vi "DAQmx_Put_Master_First.vi"(8 "error in (no error)":errorcluster, 11 "DAQmx in":refnum<class "DAQmx.lvclass">[](array[class])) -> (0 "error out":errorcluster, 3 "DAQmx out":refnum<class "DAQmx.lvclass">[](array[class]))   [LabVIEW 2020, in "DAQmx.lvclass"]
uses:
  DAQmx.lvclass
  DAQmx.lvclass/DAQmx.ctl
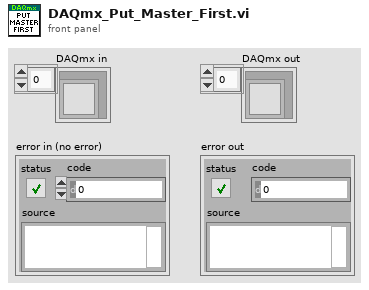
[diagram p1: front panel]
types:
  T1 = typedef "DAQmx.lvclass/DAQmx_Config.ctl" = cluster{"Buffer Size (S)":i32, "Master Slave":enum16{"MASTER", "SLAVE"}}
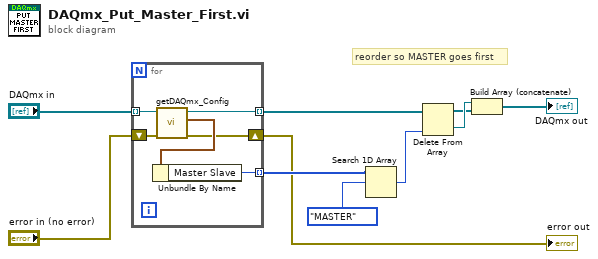
[diagram p0: block diagram]
diagram:
  # "reorder so MASTER goes first"
  n1 = for {
    tunnel: "DAQmx in" -> [w16] mode=indexing
    tunnel: [w14] -> w5 mode=indexing
    tunnel: [w13] -> w6 mode=indexing
    shift-right: [w11] -> w1
    shift-left: "error in (no error)" -> [w12]
    n2 = call "getDAQmx_Config.vi"("error in (no error)"=w12, "DAQmx in"=w16) -> ("error out"=w11:errorcluster, "DAQmx.Config"=w15:T1, "DAQmx out"=w13:refnum<class "DAQmx.lvclass">)  [unwired: 7 in]
    n3 = Unbundle By Name(w15) -> ("Master Slave"=w14:enum16{"MASTER", "SLAVE"})
  }
  "error out" <- w1
  n4 = Search 1D Array(1D array=w5, element=enum16{"MASTER", "SLAVE"}."MASTER" ("Master Slave")) -> (index of element=w3:i32)  [unwired: 1 in]
  n5 = Delete From Array(array=w6, index=w3) -> (deleted portion=w9:refnum<class "DAQmx.lvclass">, array with subset deleted=w8:refnum<class "DAQmx.lvclass">[])  [unwired: 1 in]
  n6 = Build Array (concatenate)(w9, w8) -> (→"DAQmx out":refnum<class "DAQmx.lvclass">[])
